vi "RF_Attn_query.vi"(1 "Parameter":enum16{"Attenuation (dB)"}(ring), 2 "USB address":string="0:19") -> (0 "value":dbl format="%#_24g")   [LabVIEW 2013]
uses:
  Attenuator_Vaunix-LDA_LabView_32Bit_Driver/Vaunix LDA/Vaunix LDA.lvlib
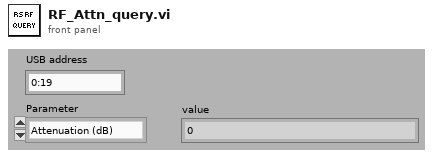
[diagram p1: front panel]
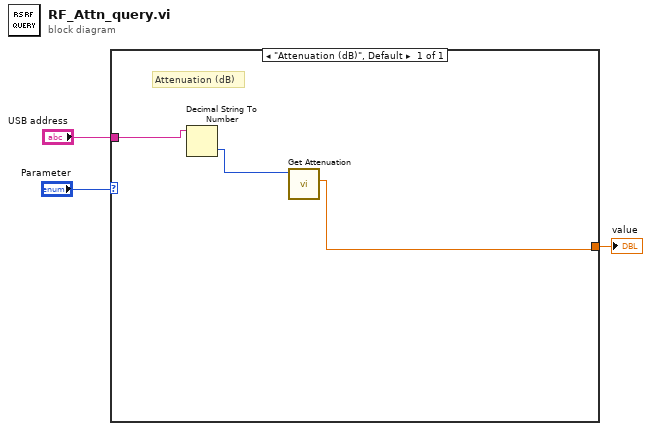
[diagram p0: block diagram]
diagram:
  n1 = case shown="\"Attenuation (dB)\", Default" "Parameter" {
    tunnel: "USB address" -> [w6]
    tunnel: [w4] -> w1
    frame "Attenuation (dB)", Default {
      # "Attenuation (dB)"
      n2 = Decimal String To Number(string=w6) -> (number=w5:i32)  [unwired: 2 in, 1 out]
      n3 = call "Get Attenuation.vi"("Device ID in"=w5) -> ("Attenuation (dB)"=w4:dbl)  [unwired: 8 in, 2 out]
    }
  }
  "value" <- w1
